vi "Core.vi"(0 "AFE_Inputs":T4, 1 "AFE_Gains":T3, 2 "AFE_Params":T6, 5 "AFE_Setpoints":T8, 7 "AFE_Ranges":T7={"PLL_PIRad_high"=inf, "PLL_PiRad_low"=inf, "IQcmd_high"=inf, "IQcmd_low"=inf, "IDcmd_high"=inf, "IDcmd_low"=inf, "VDcmd_high"=inf, "VDcmd_low"=inf, "VQmcd_high"=inf, "VQcmd_low"=inf}, 9 "input valid":bool=TRUE, 11 "AFE_ControlSignals":T9, 12 "AFE_ManualControl":T5) -> (3 "AFE_Actions":T2, 4 "AFE_Outputs":T1, 10 "output valid":bool, 15 "ready for input":bool)   [LabVIEW 2015, in "ActiveFrontEnd.lvlib"]
uses:
  ActiveFrontEnd.lvlib
  Signals.ctl
  Setpoint.ctl
  Range.ctl
  Parameters.ctl
  ManualControl.ctl
  Inputs.ctl
  Gains.ctl
  Actions.ctl
  Outputs.ctl
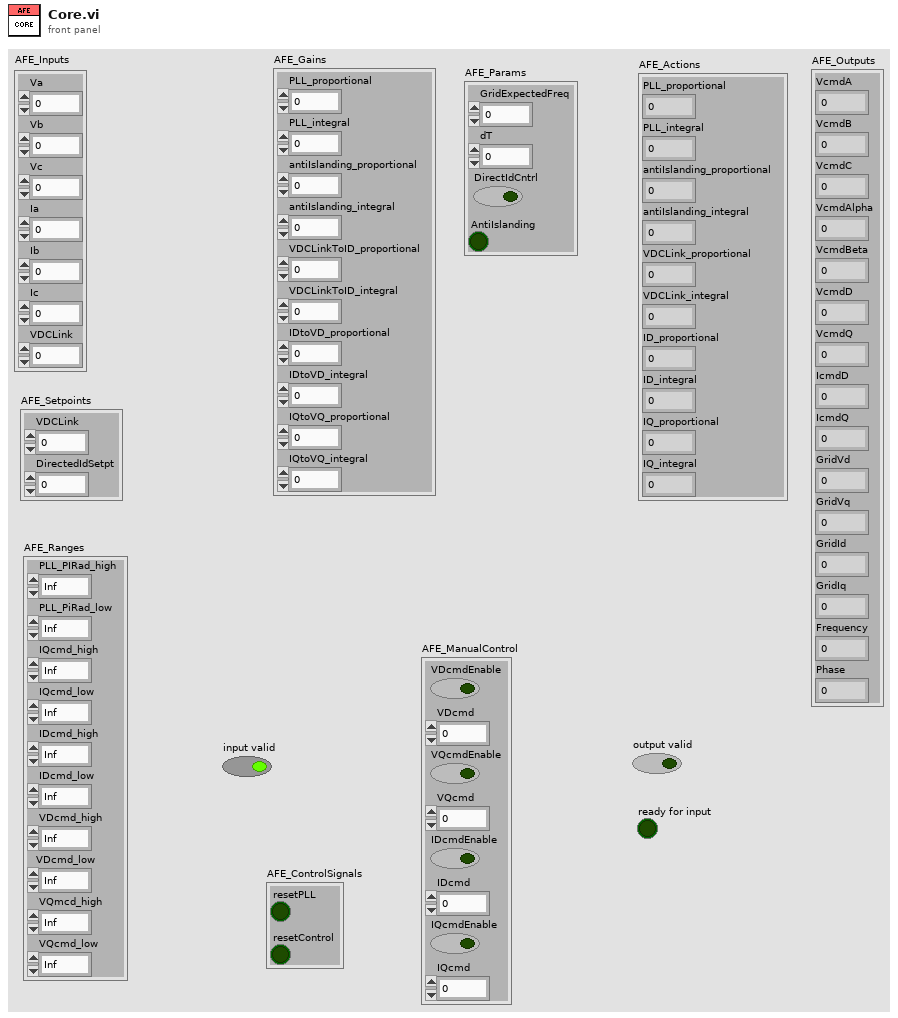
[diagram p1: front panel]
types:
  T1 = typedef "ActiveFrontEnd.lvlib/Outputs.ctl" = cluster{"VcmdA":sgl, "VcmdB":sgl, "VcmdC":sgl, "VcmdAlpha":sgl, "VcmdBeta":sgl, "VcmdD":sgl, "VcmdQ":sgl, "IcmdD":sgl, "IcmdQ":sgl, "GridVd":sgl, "GridVq":sgl, "GridId":sgl, "GridIq":sgl, "Frequency":sgl, "Phase":sgl}
  T2 = typedef "ActiveFrontEnd.lvlib/Actions.ctl" = cluster{"PLL_proportional":sgl, "PLL_integral":sgl, "antiIslanding_proportional":sgl, "antiIslanding_integral":sgl, "VDCLink_proportional":sgl, "VDCLink_integral":sgl, "ID_proportional":sgl, "ID_integral":sgl, "IQ_proportional":sgl, "IQ_integral":sgl}
  T3 = typedef "ActiveFrontEnd.lvlib/Gains.ctl" = cluster{"PLL_proportional":sgl, "PLL_integral":sgl, "antiIslanding_proportional":sgl, "antiIslanding_integral":sgl, "VDCLinkToID_proportional":sgl, "VDCLinkToID_integral":sgl, "IDtoVD_proportional":sgl, "IDtoVD_integral":sgl, "IQtoVQ_proportional":sgl, "IQtoVQ_integral":sgl}
  T4 = typedef "ActiveFrontEnd.lvlib/Inputs.ctl" = cluster{"Va":sgl, "Vb":sgl, "Vc":sgl, "Ia":sgl, "Ib":sgl, "Ic":sgl, "VDCLink":sgl}
  T5 = typedef "ActiveFrontEnd.lvlib/ManualControl.ctl" = cluster{"VDcmdEnable":bool, "VDcmd":sgl, "VQcmdEnable":bool, "VQcmd":sgl, "IDcmdEnable":bool, "IDcmd":sgl, "IQcmdEnable":bool, "IQcmd":sgl}
  T6 = typedef "ActiveFrontEnd.lvlib/Parameters.ctl" = cluster{"GridExpectedFreq":sgl, "dT":sgl, "DirectIdCntrl":bool, "AntiIslanding":bool}
  T7 = typedef "ActiveFrontEnd.lvlib/Range.ctl" = cluster{"PLL_PIRad_high":sgl, "PLL_PiRad_low":sgl, "IQcmd_high":sgl, "IQcmd_low":sgl, "IDcmd_high":sgl, "IDcmd_low":sgl, "VDcmd_high":sgl, "VDcmd_low":sgl, "VQmcd_high":sgl, "VQcmd_low":sgl}
  T8 = typedef "ActiveFrontEnd.lvlib/Setpoint.ctl" = cluster{"VDCLink":sgl, "DirectedIdSetpt":sgl}
  T9 = typedef "ActiveFrontEnd.lvlib/Signals.ctl" = cluster{"resetPLL":bool, "resetControl":bool}
  T10 = cluster{"VcmdA":sgl, "VcmdB":sgl, "VcmdC":sgl, "VcmdAlpha":sgl, "VcmdBeta":sgl, "GridVd":sgl, "GridVq":sgl, "GridId":sgl, "GridIq":sgl, "Frequency":sgl, "Phase":sgl}
  T11 = cluster{"PLL_proportional":sgl, "PLL_integral":sgl, "antiIslanding_proportional":sgl, "antiIslanding_integral":sgl, "VDCLink_proportional":sgl, "VDCLink_integral":sgl, "ID_proportional":sgl, "ID_integral":sgl, "IQ_proportional":sgl, "IQ_integral":sgl}
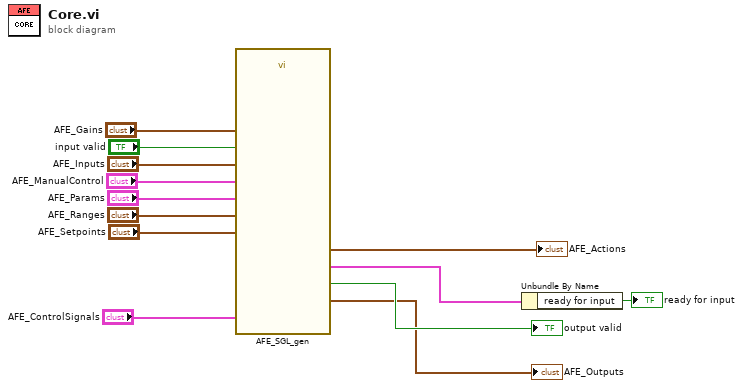
[diagram p0: block diagram]
diagram:
  n1 = call "AFE_SGL_gen.vi"("Inputs"="AFE_Inputs", "Gains"="AFE_Gains", "Range"="AFE_Ranges", "Setpoints"="AFE_Setpoints", "Signals"="AFE_ControlSignals", "input valid"="input valid", "Parameters"="AFE_Params", "ManualControl"="AFE_ManualControl") -> ("Outputs"=→"AFE_Outputs":T10, "output valid"=→"output valid":bool, "feedback signals"=w11:cluster{"ready for input":bool}, "Actions"=→"AFE_Actions":T11)  [unwired: 4 in]
  n2 = Unbundle By Name(w11) -> ("ready for input"=→"ready for input":bool)
